vi "ELVIS III v1.0 Build MUX Configuration AI IRQ.vi"(11 "IO IRQ Channels Enum":T4) -> (3 "Channel Reservation Info":T1)   [LabVIEW 2021]
uses:
  <vilib>/myRIO/Common/Instrument Driver Framework/myRIO v1.0/IRQ/typedefs/IO IRQ Channels Enum.ctl
  <vilib>/myRIO/Common/Instrument Driver Framework/ELVIS III v1.0/Resource Manager/typedefs/ELVIS III v1.0 Channel Reservation List.ctl
  <vilib>/myRIO/Common/Instrument Driver Framework/ELVIS III v1.0/Resource Manager/typedefs/ELVIS III v1.0 Channel Reservation Info.ctl
  <vilib>/myRIO/Common/Instrument Driver Framework/ELVIS III v1.0/Resource Manager/typedefs/ELVIS III v1.0 Connector List.ctl
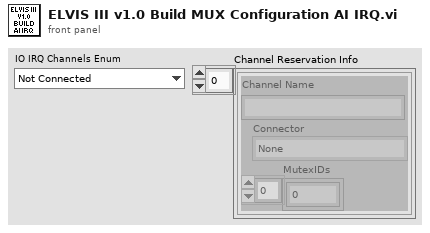
[diagram p1: front panel]
types:
  T1 = typedef "ELVIS III v1.0 Channel Reservation List.ctl" = T2[]
  T2 = typedef "ELVIS III v1.0 Channel Reservation Info.ctl" = cluster{"Channel Name":string, "Connector":T3, "MutexIDs":u32[]}
  T3 = typedef "ELVIS III v1.0 Connector List.ctl" = enum32{"None", "ConnectorA", "ConnectorB"}
  T4 = typedef "IO IRQ Channels Enum.ctl" = enum16{"Not Connected", "A/AI0 (Interrupt)", "A/AI1 (Interrupt)", "A/DIO0 (Interrupt)", "A/DIO1 (Interrupt)", "A/DIO2 (Interrupt)", "A/DIO3 (Interrupt)", "Button0 (Interrupt)", "B/AI0 (Interrupt)", "B/AI1 (Interrupt)", "B/DIO0 (Interrupt)", "B/DIO1 (Interrupt)", "B/DIO2 (Interrupt)", "B/DIO3 (Interrupt)"}
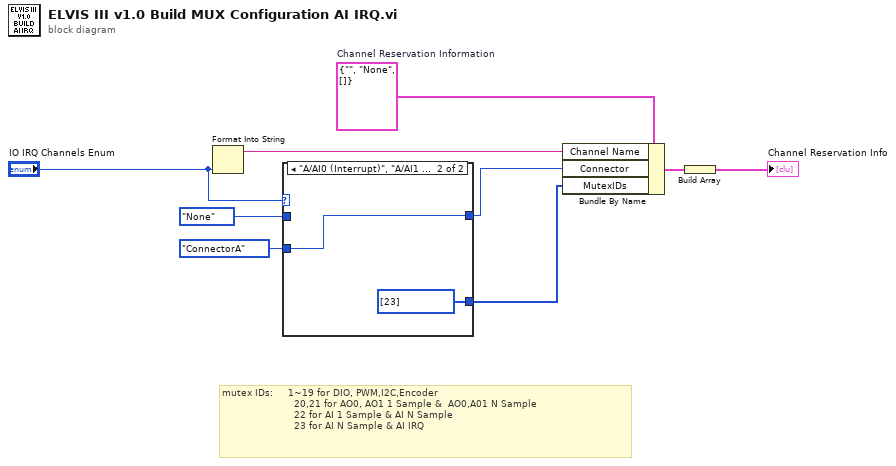
[diagram p0: block diagram]
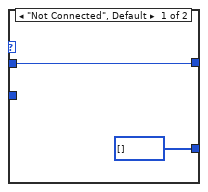
[diagram p2: hidden frame]
diagram:
  w8 = T2 {"Channel Name"="", "Connector"=enum."None", "MutexIDs"=[]}  # Channel Reservation Information
  # "mutex IDs:     1~19 for DIO, PWM,I2C,Encoder\n                        20,21 for AO0, AO1 1 Sample &  AO0,A01 N Sample\n                        22 for AI 1 Sample & AI N Sample\n                        23 for AI N Sample & AI IRQ"
  n1 = Format Into String("IO IRQ Channels Enum") -> (resulting string=w7:string)  [unwired: 3 in, 1 out]
  n2 = case shown="\"A/AI0 (Interrupt)\", \"A/AI1 (Interrupt)\"" "IO IRQ Channels Enum" {
    tunnel: [u32[] [] ("MutexIDs") u32[] [23] ("MutexIDs")] -> w6
    tunnel: ELVIS_III_v1.0_Connector_List."None" ("Connector") -> [w11 _]
    tunnel: [w11 w13] -> w4
    tunnel: ELVIS_III_v1.0_Connector_List."ConnectorA" ("Connector") -> [_ w13]
    frame "Not Connected", Default {
    }
    frame "A/AI0 (Interrupt)", "A/AI1 (Interrupt)" {
    }
  }
  n3 = Bundle By Name(cluster=w8, "Channel Name"=w7, "Connector"=w4, "MutexIDs"=w6) -> (w2:T2)
  n4 = Build Array(w2) -> (→"Channel Reservation Info":T2[])
